vi "Login.vi"(8 "error in (no error)":errorcluster) -> (0 "error out":errorcluster)   [LabVIEW 2017]
uses:
  <vilib>/addons/database/Connection.llb/DB Tools Open Connec (Path).vi
  Globle/Trigger Home Screen.vi
  Globle/Login Data.vi
  Globle/Login Details.vi
  <vilib>/addons/database/NI_Database_API.lvlib
panel:
  in  "Cancel Button - Archive":bool
  in  "Authority":string(combo)
  in  "Username":string(combo)
  in  "Password":string
  in  "Login":bool
  in  "Cancel":bool
  # "User Login"
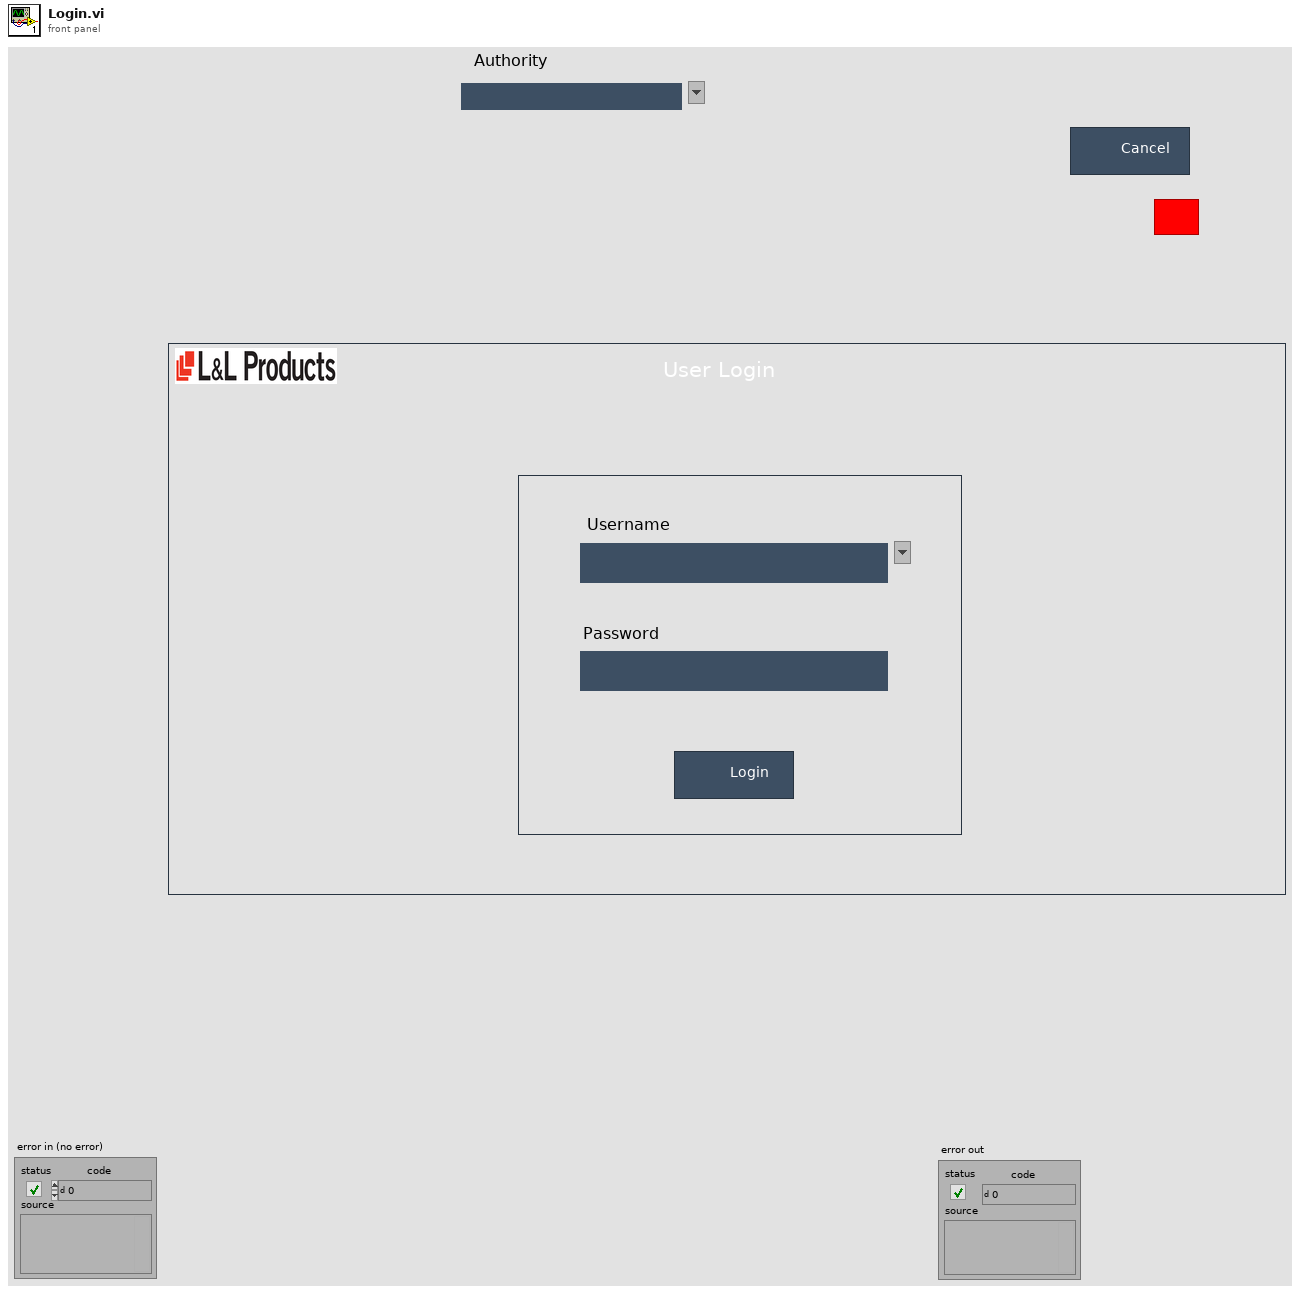
[diagram p1: front panel]
types:
  T1 = typedef "NI_Database_API.lvlib/Conn ObjectReference.ctl" = refnum<k1>
  T2 = cluster{"SCREEN 1":bool, "SCREEN 2":bool, "SCREEN 3":bool, "SCREEN 4":bool, "SCREEN 5":bool, "SCREEN 6":bool, "SCREEN 7":bool, "SCREEN 8":bool, "SCREEN 9":bool, "SCREEN 10":bool, "SCREEN 11":bool, "SCREEN 12":bool, "SCREEN 13":bool, "SCREEN 14":bool, "SCREEN 15":bool, "SCREEN 16":bool, "SCREEN 17":bool, "SCREEN 18":bool, "SCREEN 19":bool, "SCREEN 20":bool}
  T3 = enum32{"invalid app kind", "Development System", "Run Time System", "Student Edition", "Embedded LabVIEW", "Evaluation", "Custom"}
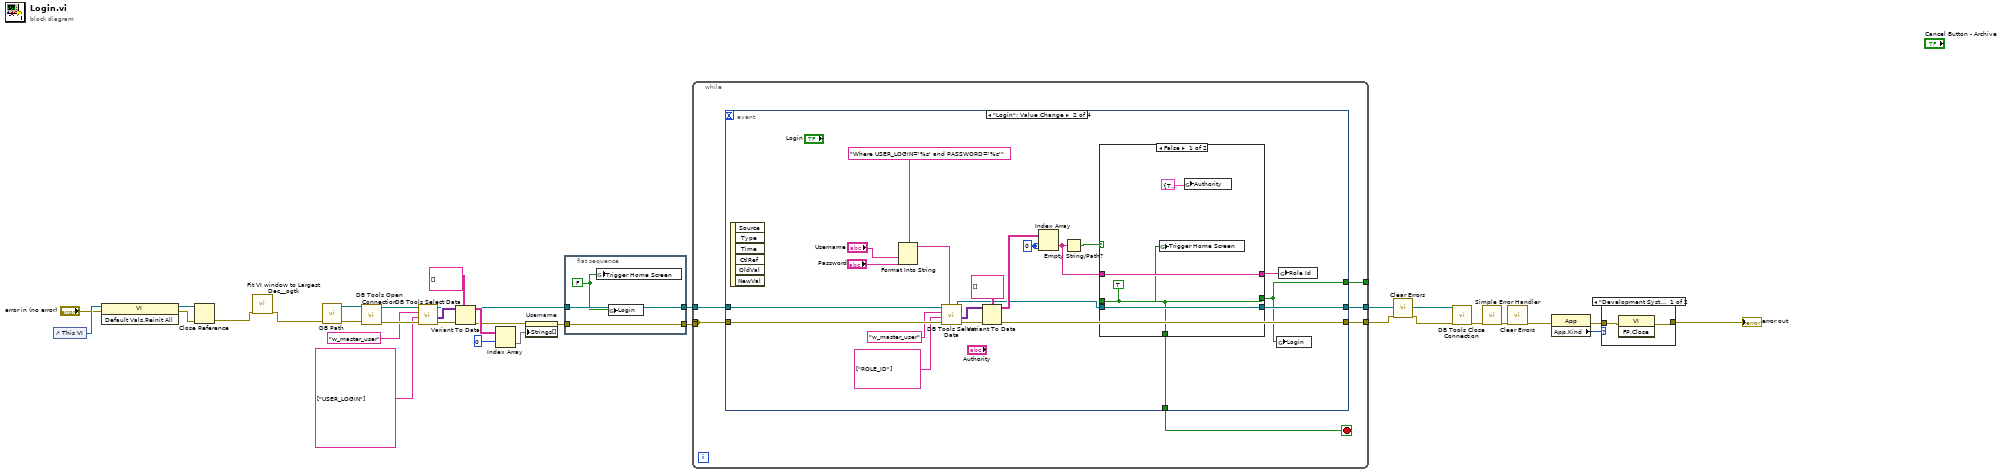
[diagram p0: block diagram]
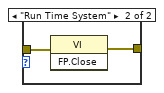
[diagram p2: hidden frame]
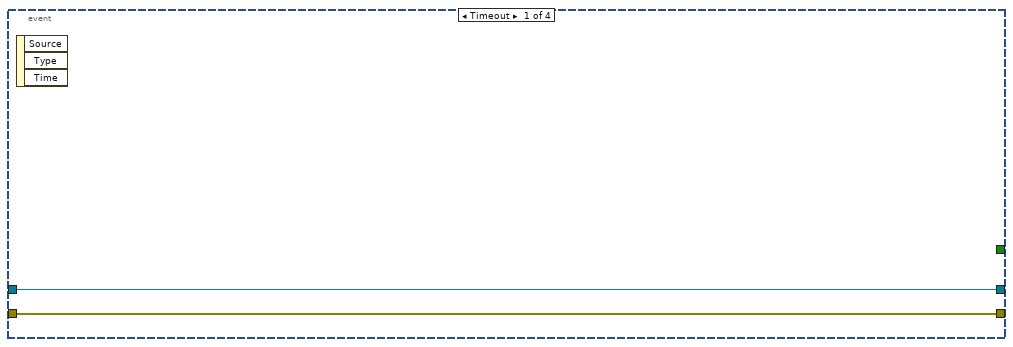
[diagram p3: hidden frame]
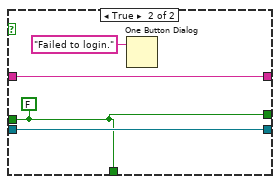
[diagram p4: hidden frame]
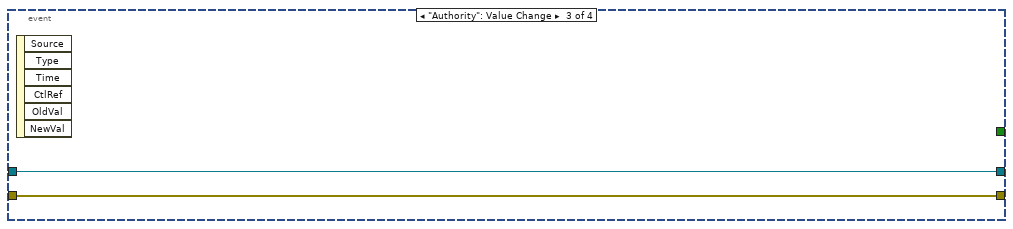
[diagram p5: hidden frame]
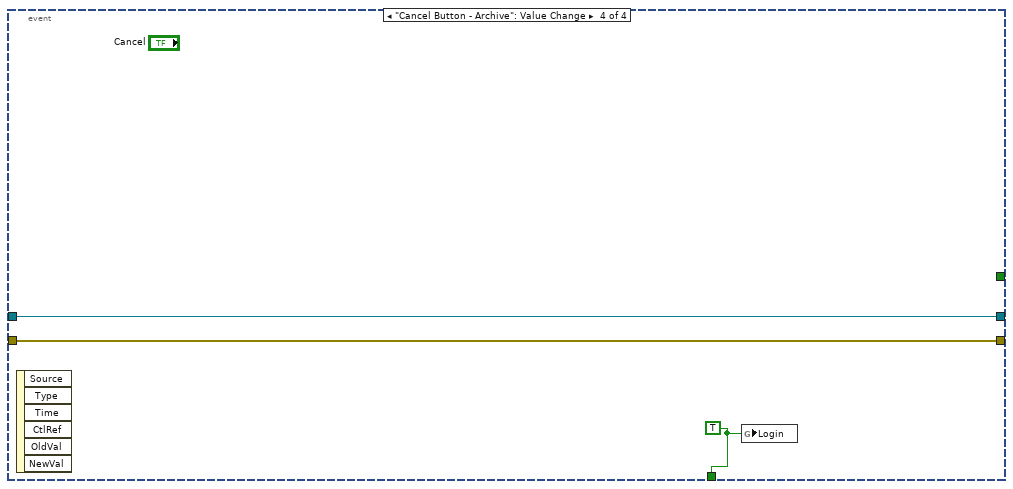
[diagram p6: hidden frame]
diagram:
  n1 = control-ref of="This VI"() -> (w32:refnum<vi>)
  n2 = invoke class="VI" method="Default Vals.Reinit All"(reference=w32, error in="error in (no error)") -> (reference out=w31:refnum<vi>, error out=w30:errorcluster)  [unwired: 1 in, 1 out]
  n3 = Close Reference(reference=w31, error in (no error)=w30) -> (error out=w2:errorcluster)
  n4 = call <userlib>:"Fit VI window to Largest Dec__ogtk.vi"("error in (no error)"=w2) -> ("error out"=w1:errorcluster)  [unwired: 5 in, 1 out]
  n5 = call "DB Path.vi"("error in"=w1) -> ("error out"=w29:errorcluster, "DB Path"=w28:path)  [unwired: 9 in]
  n6 = call-poly <vilib>:"DB Tools Open Connection.vi"("error in (no error)"=w29, "connection information"=w28) -> ("error out"=w27:errorcluster, "connection reference"=w26:T1)  [unwired: 6 in]
  n7 = call <vilib>:"DB Tools Select Data.vi"("error in (no error)"=w27, "columns"=string[] ["USER_LOGIN"], "table"="w_master_user", "connection reference"=w26) -> ("error out"=w19:errorcluster, "data"=w18:variant[][], "connection reference out"=w11:T1)  [unwired: 2 in]
  n8 = Variant To Data(error in=w19, type=string[][] [], Variant=w18) -> (data=w16:string[][], error out=w13:errorcluster)
  n9 = Index Array(array=w16, index (col)=0 ("disabled index (col)")) -> (element=w14:string[])  [unwired: 1 in]
  n10 = property on="Username" class="CmbBox"(error in=w13, "Strings[]"=w14) -> (error out=w9:errorcluster)  [unwired: 1 in, 1 out]
  n11 = flat-sequence {
    tunnel: w11 -> [w35]
    tunnel: [w35] -> w10
    tunnel: w9 -> [w34]
    tunnel: [w34] -> w8
    frame #0 {
      w33 = FALSE ("Login")
      n12 = global write "Trigger Home Screen.vi" "Trigger Home Screen"(w33) -> ()
      n13 = global write "Login Data.vi" "Login"(w33) -> ()
    }
  }
  n14 = while {
    tunnel: [w37] -> _
    tunnel: [w41] -> w5
    tunnel: w10 -> [w40]
    tunnel: [w38] -> w12
    tunnel: w8 -> [w37]
    tunnel: [w36] -> _
    stop <- w39 stop-if-true
    n15 = event shown="[1] \"Login\": Value Change" {
      selector: _ -> [_ _ _ _]
      dyn-events: _ -> [_ _ _ _]
      timeout: _ -> [_ _ _ _]
      tunnel: w37 -> [w43 w61 w73 w77]
      tunnel: [w43 w46 w73 w77] -> w41
      tunnel: w40 -> [w42 w59 w74 w76]
      tunnel: [_ w50 _ w75] -> w39
      tunnel: [w42 w47 w74 w76] -> w38
      tunnel: [_ w45 _ _] -> w36
      event Timeout {
        n16 = event-data() -> ()  [unwired: 1 in, 3 out]
      }
      event "Login": Value Change {
        w52 = 0 ("index (row)")
        n17 = event-data() -> ()  [unwired: 1 in, 6 out]
        n18 = Format Into String(format string="Where USER_LOGIN='%s' and PASSWORD='%s'", "Username", "Password") -> (resulting string=w60:string)  [unwired: 2 in, 1 out]
        n19 = call <vilib>:"DB Tools Select Data.vi"("condition"=w60, "error in (no error)"=w61, "columns"=string[] ["ROLE_ID"], "table"="w_master_user", "connection reference"=w59) -> ("error out"=w55:errorcluster, "data"=w56:variant[][], "connection reference out"=w48:T1)  [unwired: 1 in]
        n20 = Variant To Data(error in=w55, type=string[][] [], Variant=w56) -> (data=w53:string[][], error out=w46:errorcluster)
        n21 = Index Array(array=w53, index (row)=w52, index (col)=w52) -> (element=w49:string)
        n22 = Empty String/Path?(string/path=w49) -> (empty?=w51:bool)
        n23 = case shown="False" w51 {
          tunnel: [w66 w69] -> w50
          tunnel: w49 -> [w68 w71]
          tunnel: [w68 w71] -> w44
          tunnel: w48 -> [w67 w70]
          tunnel: [w67 w70] -> w47
          tunnel: [w66 w69] -> w45
          tunnel: [w66 w69] -> _
          frame False {
            w66 = TRUE
            n24 = global write "Trigger Home Screen.vi" "Trigger Home Screen"(w66) -> ()
            n25 = global write "Login Details.vi" "Authority"(T2 {"SCREEN 1"=TRUE, "SCREEN 2"=TRUE, "SCREEN 3"=TRUE, "SCREEN 4"=TRUE, "SCREEN 5"=TRUE, "SCREEN 6"=TRUE, "SCREEN 7"=TRUE, "SCREEN 8"=TRUE, "SCREEN 9"=TRUE, "SCREEN 10"=TRUE, "SCREEN 11"=TRUE, "SCREEN 12"=TRUE, "SCREEN 13"=TRUE, "SCREEN 14"=TRUE, "SCREEN 15"=TRUE, "SCREEN 16"=TRUE, "SCREEN 17"=TRUE, "SCREEN 18"=TRUE, "SCREEN 19"=TRUE, "SCREEN 20"=TRUE} ("Authority")) -> ()
          }
          frame True {
            w69 = FALSE
            n26 = One Button Dialog(message="Failed to login.") -> ()  [unwired: 1 in, 1 out]
          }
        }
        n27 = global write "Login Data.vi" "Login"(w45) -> ()
        n28 = global write "Login Data.vi" "Role Id"(w44) -> ()
      }
      event "Authority": Value Change {
        n29 = event-data() -> ()  [unwired: 1 in, 6 out]
      }
      event "Cancel Button - Archive": Value Change {
        w75 = TRUE
        n30 = event-data() -> ()  [unwired: 1 in, 6 out]
        n31 = global write "Login Data.vi" "Login"(w75) -> ()
      }
    }
  }
  n32 = call <vilib>:"Clear Errors.vi"("error in (no error)"=w5) -> ("error out"=w4:errorcluster)  [unwired: 5 in, 1 out]
  n33 = call <vilib>:"DB Tools Close Connection.vi"("error in (no error)"=w4, "connection reference"=w12) -> ("error out"=w25:errorcluster)  [unwired: 5 in]
  n34 = call <vilib>:"Simple Error Handler.vi"("error in (no error)"=w25) -> ("error out"=w24:errorcluster)  [unwired: 4 in, 4 out]
  n35 = call <vilib>:"Clear Errors.vi"("error in (no error)"=w24) -> ("error out"=w3:errorcluster)  [unwired: 5 in, 1 out]
  n36 = property class="App"(error in=w3) -> (error out=w23:errorcluster, "App.Kind"=w22:T3)  [unwired: 1 in, 1 out]
  n37 = case shown="\"Development System\", Default" w22 {
    tunnel: w23 -> [w79 w81]
    tunnel: [w78 w80] -> w7
    frame "Development System", Default {
      n38 = invoke class="VI" method="FP.Close"(error in=w79) -> (error out=w78:errorcluster)  [unwired: 2 in, 2 out]
    }
    frame "Run Time System" {
      n39 = invoke class="VI" method="FP.Close"(error in=w81) -> (error out=w80:errorcluster)  [unwired: 2 in, 2 out]
    }
  }
  "error out" <- w7
